vi "Update Variable List.vi"(4 "Data Type":T1(ring), 6 "Value":variant, 8 "error in (no error)":errorcluster, 9 "Time Stamp":timestamp, 10 "Shared Variable":refnum<k21>, 11 "Value List Reference In":refnum<vi>) -> (0 "error out":errorcluster, 3 "Value List Reference Out":refnum<vi>)   [LabVIEW 2024]
doc: "Updates the variable list in the subsystem view."
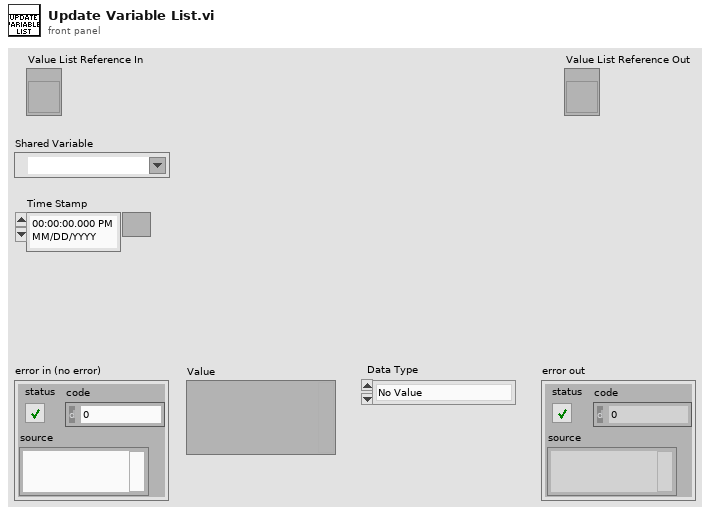
[diagram p1: front panel]
types:
  T1 = enum16{"No Value", "Custom", "Double", "Boolean", "U32", "String", "DBL Array", "I32 Array", "I32", "SGL Array", "SGL", "I8", "U8", "I16", "U16", "I64", "U64", "DBL Waveform", "I16 Waveform", "Boolean Array", "I8 Array", "U8 Array", "I16 Array", "U16 Array", "U32 Array", "I64 Array", "U64 Array", "DBL Waveform Array", "I16 Waveform Array"}
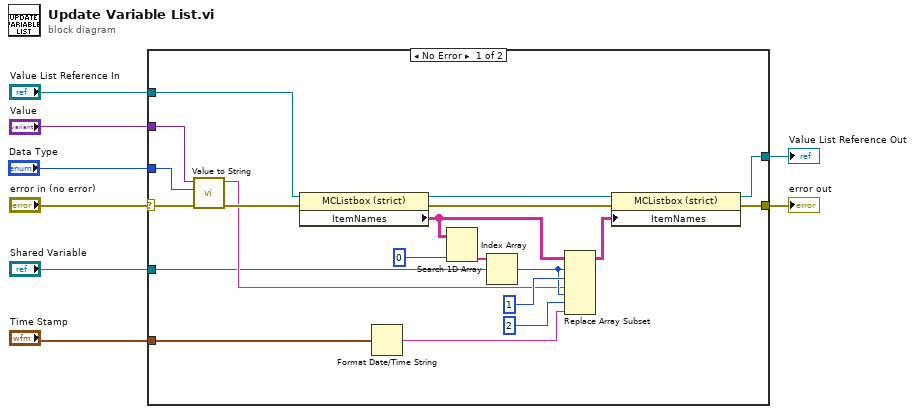
[diagram p0: block diagram]
diagram:
  n1 = case shown="No Error" "error in (no error)" {
    selector: "error in (no error)" -> [w13 w30]
    tunnel: [w17 w30] -> w7
    tunnel: "Time Stamp" -> [w16 _]
    tunnel: "Data Type" -> [w21 _]
    tunnel: "Value" -> [w20 _]
    tunnel: "Shared Variable" -> [w11 _]
    tunnel: "Value List Reference In" -> [w19 w29]
    tunnel: [w18 w29] -> w2
    frame No Error {
      n2 = call "Value to String.vi"("error in (no error)"=w13, "Data Type"=w21, "Value"=w20) -> ("error out"=w14:errorcluster, "Value String"=w12:string)  [unwired: 7 in]
      n3 = property on="Property Node" class="MCListbox (strict)"(reference=w19, error in=w14) -> (reference out=w23:refnum<vi>, error out=w24:errorcluster, "ItemNames"=w9:string[][])
      n4 = Format Date/Time String(seconds (now)=w16) -> (date/time string=w15:string)  [unwired: 2 in]
      n5 = Index Array(array=w9, index (col)=0 ("disabled index (col)")) -> (element=w28:string[])  [unwired: 1 in]
      n6 = Search 1D Array(1D array=w28, element=w11) -> (index of element=w25:i32)  [unwired: 1 out]
      n7 = Replace Array Subset(array=w9, new element #1=w12, index (row) #1=w25, index (col) #1=1 ("disabled index (row)"), new element #2=w15, index (row) #2=w25, index (col) #2=2 ("index (col)")) -> (w22:string[][])
      n8 = property on="Property Node" class="MCListbox (strict)"(reference=w23, error in=w24, "ItemNames"=w22) -> (reference out=w18:refnum<vi>, error out=w17:errorcluster)
    }
    frame Error {
    }
  }
  "error out" <- w7
  "Value List Reference Out" <- w2
